vi "Close.vi"(8 "error in (no error)":errorcluster, 11 "PythonWrapper in":refnum<class "PythonWrapper.lvclass">) -> (0 "error out":errorcluster)   [LabVIEW 2022 SP3, in "PythonWrapper.lvlib" / "PythonWrapper.lvclass"]
uses:
  PythonWrapper.lvclass
  PythonWrapper.lvclass/PythonWrapper.ctl
  PythonSession/PythonSession.lvclass
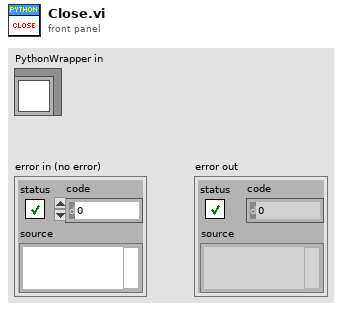
[diagram p1: front panel]
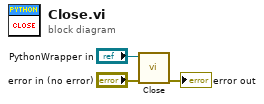
[diagram p0: block diagram]
diagram:
  n1 = call-parent "Close.vi"("error in (no error)"="error in (no error)", "PythonSession in"="PythonWrapper in") -> ("error out"=→"error out":errorcluster)  [unwired: 9 in]
